vi "CodigoLabView 2_4.vi"() -> ()   [LabVIEW 2025]
uses:
  <vilib>/Utility/NIReport.llb/Report Type.ctl
  <vilib>/Instr/_visa.llb/VISA Configure Serial Port (Instr).vi
  <vilib>/addons/_office/excel.llb/Excel Easy Table (str).vi
  <vilib>/Utility/NIReport.llb/NI_report.lvclass
  <vilib>/Utility/NIReport.llb/NI_ReportGenerationCore.lvlib
  <vilib>/addons/_office/NI_ReportGenerationToolkit.lvlib
  <vilib>/Utility/NIReport.llb/Excel/NI_Excel.lvclass
panel:
  in  "template (empty)":path
  out "Tensión":string
  out "Rele 4":bool
  out "Estado 4":string
  out "Rele 3":bool
  out "Estado 3":string
  out "Rele 2":bool
  out "Estado 2":string
  out "rele 4":string
  in  "Relé N°4":bool
  out "rele 3":string
  in  "Relé N°3":bool
  out "rele 2":string
  in  "Relé N°2":bool
  out "Estado 1":string
  out "rele 1":string
  out "Rele 1":bool
  in  "Relé N°1":bool
  out "Serial Settings":u32
  out "error out 2":errorcluster
  out "Enviando":string
  out "error out":errorcluster
  in  "VISA resource name":refnum<visa-resource-name>
  in  "stop":bool
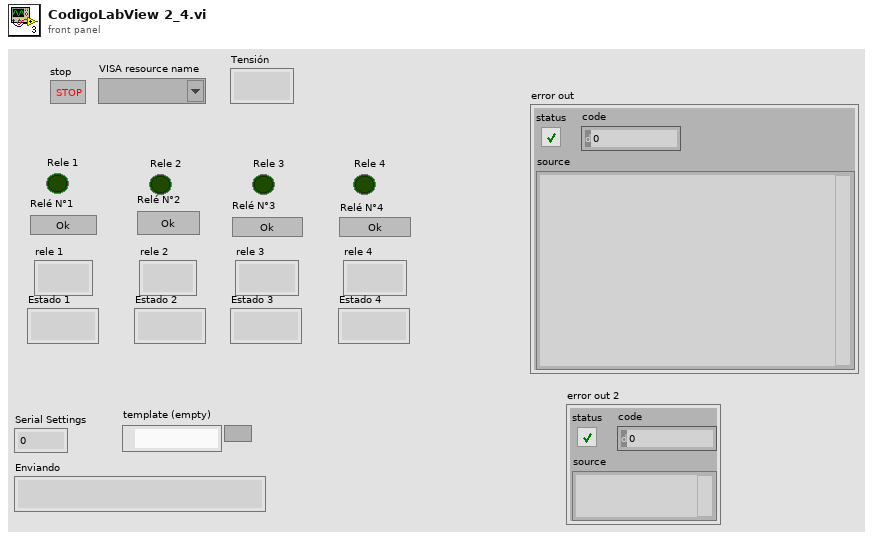
[diagram p1: front panel]
types:
  T1 = cluster{"W1":string, "W2":string, "W3":string, "W4":string, "V":string}
  T2 = typedef "NI_ReportGenerationCore.lvlib/Report Type.ctl" = enum16{"HTML", "Word", "Excel"}
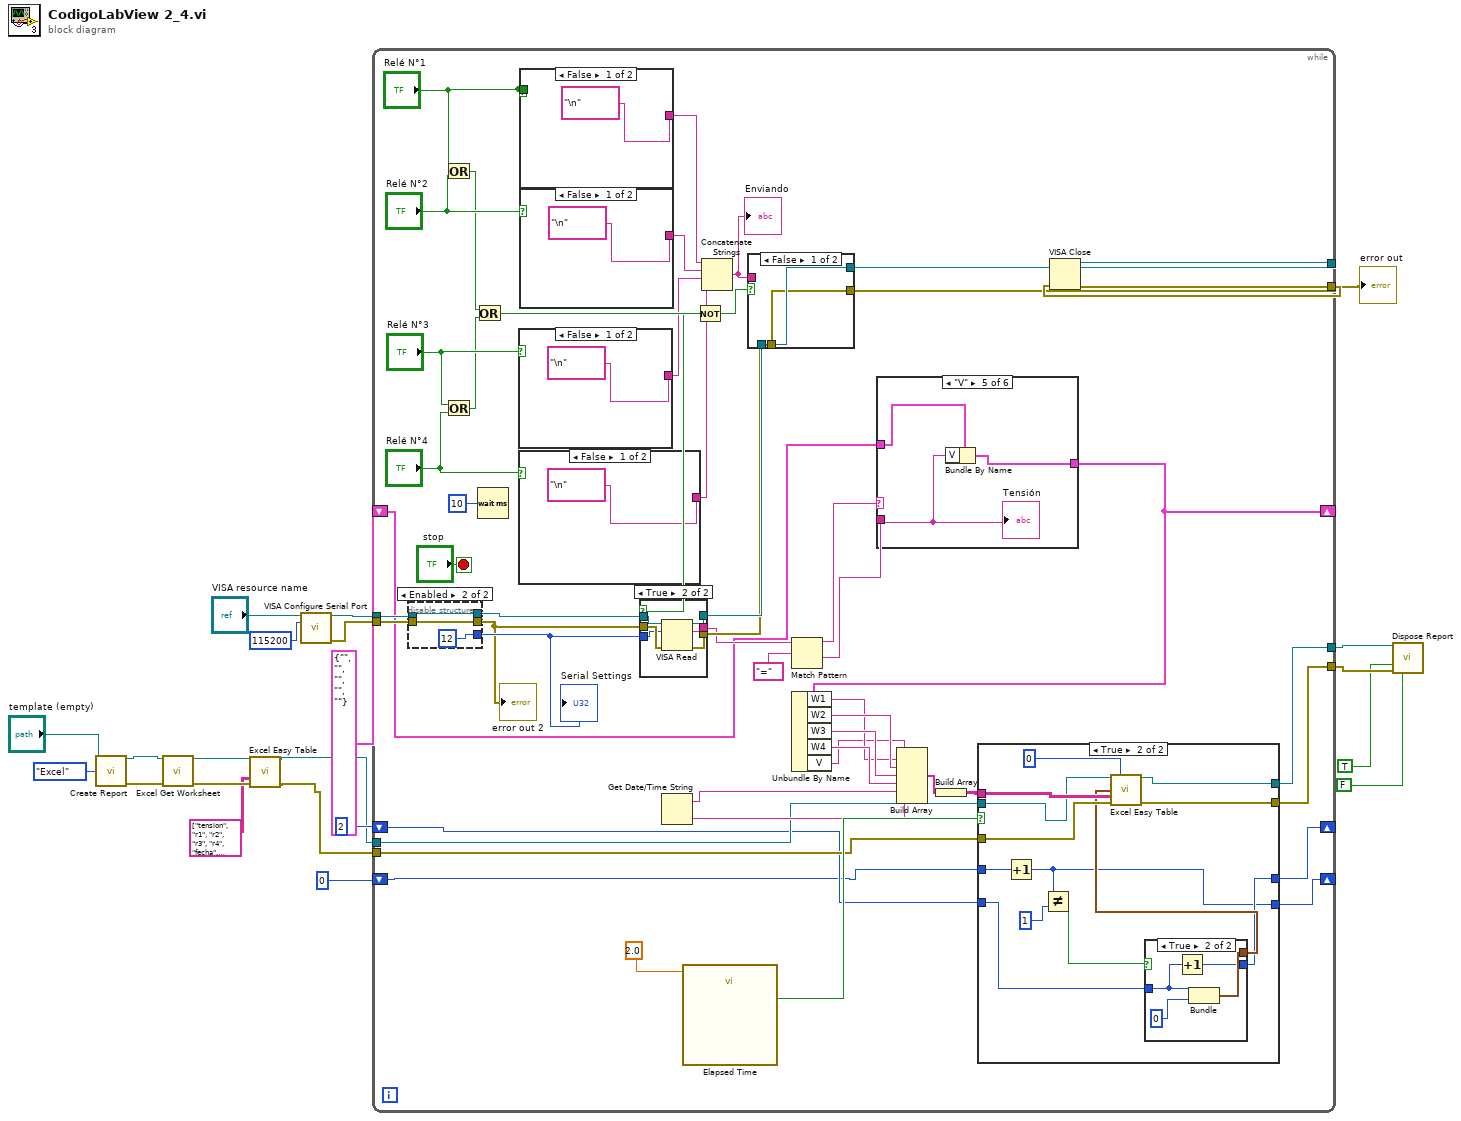
[diagram p0: block diagram]
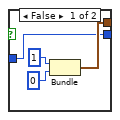
[diagram p3: hidden frame]
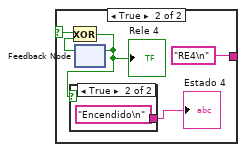
[diagram p4: hidden frame]
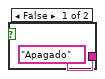
[diagram p5: hidden frame]
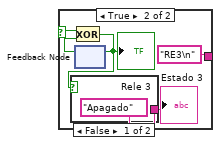
[diagram p6: hidden frame]
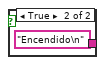
[diagram p7: hidden frame]
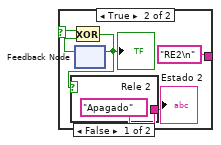
[diagram p8: hidden frame]
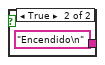
[diagram p9: hidden frame]
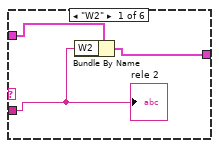
[diagram p10: hidden frame]
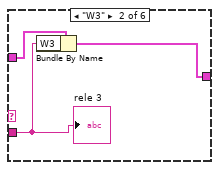
[diagram p11: hidden frame]
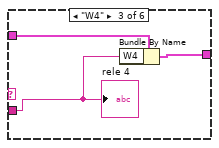
[diagram p12: hidden frame]
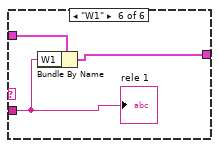
[diagram p14: hidden frame]
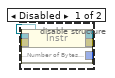
[diagram p15: hidden frame]
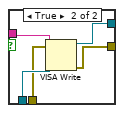
[diagram p17: hidden frame]
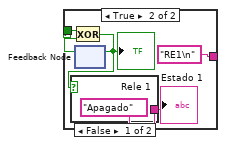
[diagram p18: hidden frame]
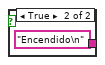
[diagram p19: hidden frame]
diagram:
  n1 = call <vilib>:"Create Report.vi"("report type"=Report_Type."Excel", "template (empty)"="template (empty)") -> ("report out"=w10:refnum<class "NI_report.lvclass">, "error out"=w9:errorcluster)  [unwired: 12 in]
  n2 = call <vilib>:"Excel Get Worksheet.vi"("report in"=w10, "error in (no error)"=w9) -> ("report out"=w4:refnum<class "NI_report.lvclass">, "error out"=w3:errorcluster)  [unwired: 12 in]
  n3 = call-poly <vilib>:"Excel Easy Table.vi"("report in"=w4, "text data"=string[][] [["tension", "r1", "r2", "r3", "r4", "fecha", "hora"]], "error in (no error)"=w3) -> ("report out"=w5:refnum<class "NI_report.lvclass">, "error out"=w6:errorcluster)  [unwired: 8 in, 3 out]
  n4 = call-poly "VISA Configure Serial Port"("VISA resource name"="VISA resource name", "baud rate (9600)"=u32 115200) -> ("VISA resource name out"=w23:refnum<visa-resource-name>, "error out"=w17:errorcluster)  [unwired: 12 in]
  n5 = while {
    tunnel: w23 -> [w71]
    tunnel: [w69] -> w22
    tunnel: w17 -> [w70]
    tunnel: [w68] -> w21
    tunnel: [w45] -> w14
    tunnel: [w44] -> w13
    tunnel: w5 -> [w38]
    tunnel: w6 -> [w37]
    shift-right: [w35] -> _
    shift-left: 2 -> [w36]
    shift-right: [w33] -> _
    shift-left: 0 -> [w34]
    shift-right: [w25] -> _
    shift-left: T1 {"W1"="", "W2"="", "W3"="", "W4"="", "V"=""} -> [w30]
    stop <- "stop" stop-if-true
    n6 = disable-structure shown="Enabled" {
      disable-tunnel: w71 -> [w142 w145]
      disable-tunnel: w70 -> [w141 w144]
      disable-tunnel: [w140 w145] -> w65
      disable-tunnel: [w139 u32 12 ("Bytes at Port")] -> w64
      disable-tunnel: [w138 w144] -> w63
      frame Disabled {
        n7 = property class="Instr"(reference=w142, error in=w141) -> (reference out=w140:refnum<visa-resource-name>, error out=w138:errorcluster, "Serial Settings:Number of Bytes at Serial Port"=w139:u32)
      }
      frame Enabled {
      }
    }
    "error out 2" <- w63
    "Serial Settings" <- w64
    n8 = Or(x="Relé N°1", y="Relé N°2") -> (x .or. y?=w54:bool)
    n9 = Or(x="Relé N°3", y="Relé N°4") -> (x .or. y?=w53:bool)
    n10 = Or(x=w54, y=w53) -> (x .or. y?=w58:bool)
    n11 = Wait (ms)(milliseconds to wait=u32 10) -> ()  [unwired: 1 out]
    n12 = case shown="False" "Relé N°3" {
      selector: "Relé N°3" -> [_ w107]
      tunnel: ["\n" "RE3\n"] -> w52
      frame False {
      }
      frame True {
        n13 = feedback #1() -> (w110:bool)  [unwired: 1 in]
        n14 = Exclusive Or(1:w110, 2:w107) -> (0:w109:bool)
        "Rele 3" <- w109
        n15 = case shown="False" w109 {
          tunnel: ["Apagado" "Encendido\n"] -> w108
          frame False {
          }
          frame True {
          }
        }
        "Estado 3" <- w108
        n16 = feedback-in #1(w109) -> ()
      }
    }
    n17 = case shown="False" "Relé N°4" {
      selector: "Relé N°4" -> [_ w99]
      tunnel: ["\n" "RE4\n"] -> w51
      frame False {
      }
      frame True {
        n18 = feedback #2() -> (w102:bool)  [unwired: 1 in]
        n19 = Exclusive Or(1:w102, 2:w99) -> (0:w101:bool)
        "Rele 4" <- w101
        n20 = case shown="True" w101 {
          tunnel: ["Apagado" "Encendido\n"] -> w100
          frame False {
          }
          frame True {
          }
        }
        "Estado 4" <- w100
        n21 = feedback-in #2(w101) -> ()
      }
    }
    n22 = case shown="False" "Relé N°1" {
      tunnel: ["\n" "RE1\n"] -> w49
      tunnel: "Relé N°1" -> [_ w165]
      frame False {
      }
      frame True {
        n23 = feedback #3() -> (w164:bool)  [unwired: 1 in]
        n24 = Exclusive Or(1:w164, 2:w165) -> (0:w163:bool)
        "Rele 1" <- w163
        n25 = case shown="False" w163 {
          tunnel: ["Apagado" "Encendido\n"] -> w162
          frame False {
          }
          frame True {
          }
        }
        "Estado 1" <- w162
        n26 = feedback-in #3(w163) -> ()
      }
    }
    n27 = case shown="False" "Relé N°2" {
      selector: "Relé N°2" -> [_ w115]
      tunnel: ["\n" "RE2\n"] -> w50
      frame False {
      }
      frame True {
        n28 = feedback #4() -> (w118:bool)  [unwired: 1 in]
        n29 = Exclusive Or(1:w118, 2:w115) -> (0:w117:bool)
        "Rele 2" <- w117
        n30 = case shown="False" w117 {
          tunnel: ["Apagado" "Encendido\n"] -> w116
          frame False {
          }
          frame True {
          }
        }
        "Estado 2" <- w116
        n31 = feedback-in #4(w117) -> ()
      }
    }
    n32 = Get Date/Time String() -> (date string=w40:string, time string=w39:string)  [unwired: 3 in]
    n33 = call "Elapsed Time"("Time Target (s)"=2.0) -> ("Time has Elapsed"=w41:bool)  [unwired: 11 in, 7 out]
    n34 = Not(x=w58) -> (.not. x?=w43:bool)
    n35 = case shown="True" w43 {
      tunnel: [w147 w153] -> w67
      tunnel: [w146 w152] -> w66
      tunnel: w63 -> [w146 w151]
      tunnel: w65 -> [w147 w150]
      tunnel: w64 -> [_ w149]
      tunnel: [_ w148] -> w32
      frame False {
      }
      frame True {
        n36 = VISA Read(VISA resource name=w150, byte count=w149, error in (no error)=w151) -> (VISA resource name out=w153:refnum<visa-resource-name>, read buffer=w148:string, error out=w152:errorcluster)  [unwired: 1 out]
      }
    }
    n37 = Concatenate Strings(w49, w50, w52, w51) -> (w48:string)
    "Enviando" <- w48
    n38 = case shown="False" w58 {
      tunnel: [w155 w160] -> w69
      tunnel: [w154 w159] -> w68
      tunnel: w67 -> [w155 w158]
      tunnel: w66 -> [w154 w157]
      tunnel: w48 -> [_ w156]
      frame False {
      }
      frame True {
        n39 = VISA Write(VISA resource name=w158, write buffer=w156, error in (no error)=w157) -> (VISA resource name out=w160:refnum<visa-resource-name>, error out=w159:errorcluster)  [unwired: 1 out]
      }
    }
    n40 = Match Pattern(string=w32, regular expression="=") -> (before substring=w60:string, after substring=w31:string)  [unwired: 1 in, 2 out]
    n41 = case shown="\"V\"" w60 {
      tunnel: w31 -> [w123 w126 w128 _ w134 w136]
      tunnel: w30 -> [w124 w127 w129 w131 w133 w137]
      tunnel: [w122 w125 w130 w131 w132 w135] -> w25
      frame "W2" {
        n42 = Bundle By Name(cluster=w124, "W2"=w123) -> (w122:T1)
        "rele 2" <- w123
      }
      frame "W3" {
        n43 = Bundle By Name(cluster=w127, "W3"=w126) -> (w125:T1)
        "rele 3" <- w126
      }
      frame "W4" {
        n44 = Bundle By Name(cluster=w129, "W4"=w128) -> (w130:T1)
        "rele 4" <- w128
      }
      frame "False", Default {
      }
      frame "V" {
        n45 = Bundle By Name(cluster=w133, "V"=w134) -> (w132:T1)
        "Tensión" <- w134
      }
      frame "W1" {
        n46 = Bundle By Name(cluster=w137, "W1"=w136) -> (w135:T1)
        "rele 1" <- w136
      }
    }
    n47 = Unbundle By Name(w25) -> ("W1"=w26:string, "W2"=w27:string, "W3"=w28:string, "W4"=w29:string, "V"=w24:string)
    n48 = Build Array(w24, w26, w27, w28, w29, w40, w39) -> (w47:string[])
    n49 = Build Array(w47) -> (w46:string[][])
    n50 = case shown="True" w41 {
      tunnel: w46 -> [_ w89]
      tunnel: w37 -> [w76 w88]
      tunnel: [w75 w87] -> w45
      tunnel: [w76 w86] -> w44
      tunnel: w38 -> [w75 w85]
      tunnel: w36 -> [w74 w82]
      tunnel: [w74 w81] -> w35
      tunnel: w34 -> [w73 w80]
      tunnel: [w73 w77] -> w33
      frame False {
      }
      frame True {
        n51 = Increment(x=w80) -> (x+1=w77:i32)
        n52 = Not Equal?(x=w77, y=1) -> (x != y?=w78:bool)
        n53 = case shown="True" w78 {
          tunnel: [w91 w97] -> w84
          tunnel: w82 -> [w90 w95]
          tunnel: [w90 w94] -> w81
          frame False {
            n54 = Bundle(1, 0) -> (w91:cluster{i32, i32})  [unwired: 1 in]
          }
          frame True {
            n55 = Increment(x=w95) -> (x+1=w94:i32)
            n56 = Bundle(w95, 0) -> (w97:cluster{i32, i32})  [unwired: 1 in]
          }
        }
        n57 = call-poly <vilib>:"Excel Easy Table.vi"("report in"=w85, "iteration"=0, "start (0, 0)"=w84, "text data"=w89, "error in (no error)"=w88) -> ("report out"=w87:refnum<class "NI_report.lvclass">, "error out"=w86:errorcluster)  [unwired: 6 in, 3 out]
      }
    }
  }
  n58 = VISA Close(VISA resource name=w22, error in (no error)=w21) -> (error out=→"error out":errorcluster)
  n59 = call-dynamic "Dispose Report.vi"("report in"=w14, "save changes? (F)"=TRUE, "error in (no error)"=w13, "close report? (T)"=FALSE) -> ()  [unwired: 11 in, 1 out]
